vi "MercuryiTCtest.vi"() -> ()   [LabVIEW 2015]
uses:
  <instrlib>/Mercury iXX/Public/Controls/Unit String.ctl
  <instrlib>/Mercury iXX/Public/Controls/Response String.ctl
  <instrlib>/Mercury iXX/Public/Controls/Comms Transport Layer.ctl
  <instrlib>/Mercury iXX/Public/Libraries/System/Open/Open System.vi
  <instrlib>/Mercury iXX/Public/Libraries/Temperature/Open/Open Temperature Device.vi
  <instrlib>/Mercury iXX/Public/Libraries/Temperature/Signals/Read/Temperature (Read).vi
  <instrlib>/Mercury iXX/Public/Libraries/Control Loop/Configuration/Set/Heater Auto (Set).vi
  <instrlib>/Mercury iXX/Mercury iXX.lvlib
  <instrlib>/Mercury iXX/Public/Libraries/System.lvlib
  <instrlib>/Mercury iXX/Public/Libraries/Temperature.lvlib
  <instrlib>/Mercury iXX/Public/Libraries/Control Loop.lvlib
panel:
  in  "Temperature setpoint":dbl=296.0 format="%#_13g"
  out "Response":T1
  out "Unit":T2
  out "Temperature":dbl
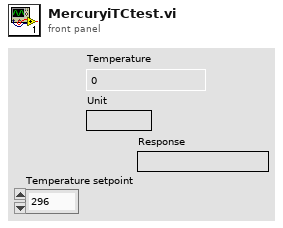
[diagram p1: front panel]
types:
  T1 = typedef "Mercury iXX.lvlib/Response String.ctl" = string
  T2 = typedef "Mercury iXX.lvlib/Unit String.ctl" = string
  T3 = typedef "Mercury iXX.lvlib/Comms Transport Layer.ctl" = enum16{"Ethernet TCP/IP", "USB", "ISOBus - RS-232", "GPIB"}
  T4 = typedef "Mercury iXX.lvlib/Mercury Reference.ctl" = cluster{"Comms":refnum<visa-resource-name>, "Device ID":string[], "Comms Layer":T3, "Command":string, "Query reference":T5}
  T5 = typedef "Mercury iXX.lvlib/Query Dynamic Reference.ctl" = refnum<vi>
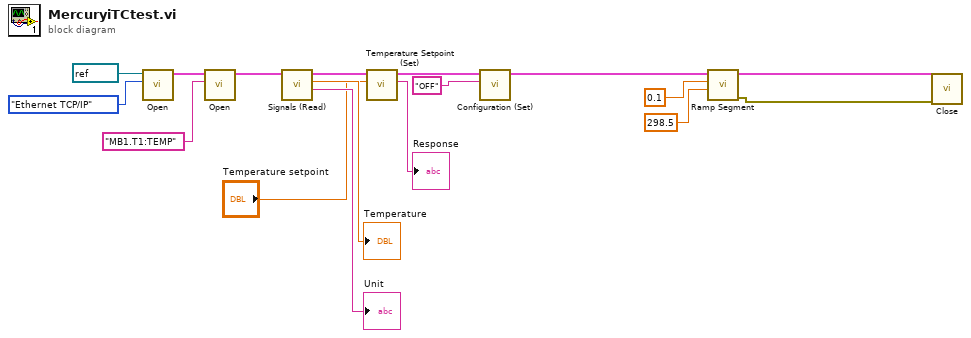
[diagram p0: block diagram]
diagram:
  n1 = call-poly <instrlib>:"Open.vi"("Comms Layer"=Comms_Transport_Layer."Ethernet TCP/IP", "VISA resource name"=refnum<visa-resource-name> "iTC") -> ("Mercury Reference Out"=w13:T4)  [unwired: 5 in, 4 out]
  n2 = call-poly <instrlib>:"Open.vi"("Device Identifier"="MB1.T1:TEMP", "Mercury Reference In"=w13) -> ("Mercury Reference Out"=w12:T4)  [unwired: 8 in, 1 out]
  n3 = call-poly <instrlib>:"Signals (Read).vi"("Mercury Reference In"=w12) -> ("Unit"=→"Unit":T2, "Temperature"=→"Temperature":dbl, "Mercury Reference Out"=w10:T4)  [unwired: 6 in, 2 out]
  n4 = call <instrlib>:"Temperature Setpoint (Set).vi"("Temperature setpoint"="Temperature setpoint", "Mercury Reference In"=w10) -> ("Response"=→"Response":T1, "Mercury Reference Out"=w7:T4)  [unwired: 6 in, 2 out]
  n5 = call-poly <instrlib>:"Configuration (Set).vi"("Heater Auto"="OFF", "Mercury Reference In"=w7) -> ("Mercury Reference Out"=w6:T4)  [unwired: 6 in, 3 out]
  n6 = call <userlib>:"Ramp Segment.vi"("Temperature setpoint"=298.5, "Ramp rate"=0.1, "Mercury Reference In"=w6) -> ("error out"=w1:errorcluster, "Mercury Reference Out"=w4:T4)  [unwired: 7 in]
  n7 = call <instrlib>:"Close.vi"("error in (no error)"=w1, "Mercury Reference"=w4) -> ()  [unwired: 9 in, 1 out]
